vi "Update En Face Array.vi"(7 "State":T1, 8 "Error In":errorcluster, 9 "A-Scans Per B-Scan":u32, 10 "Number Of BScans":u32, 11 "Slice":sgl[](array[numeric])) -> (0 "Error Out":errorcluster, 2 "B-Scan Index":i32, 3 "Array out":sgl[][](array[numeric]))   [LabVIEW 2015, in "Intensity Processing.lvclass"]
uses:
  Intensity/Intensity Processing.lvclass
  En Face States.ctl
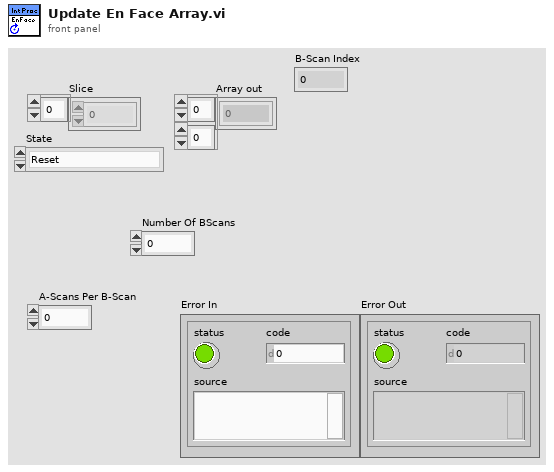
[diagram p1: front panel]
types:
  T1 = typedef "En Face States.ctl" = enum16{"Reset", "Update", "Get EnFace"}
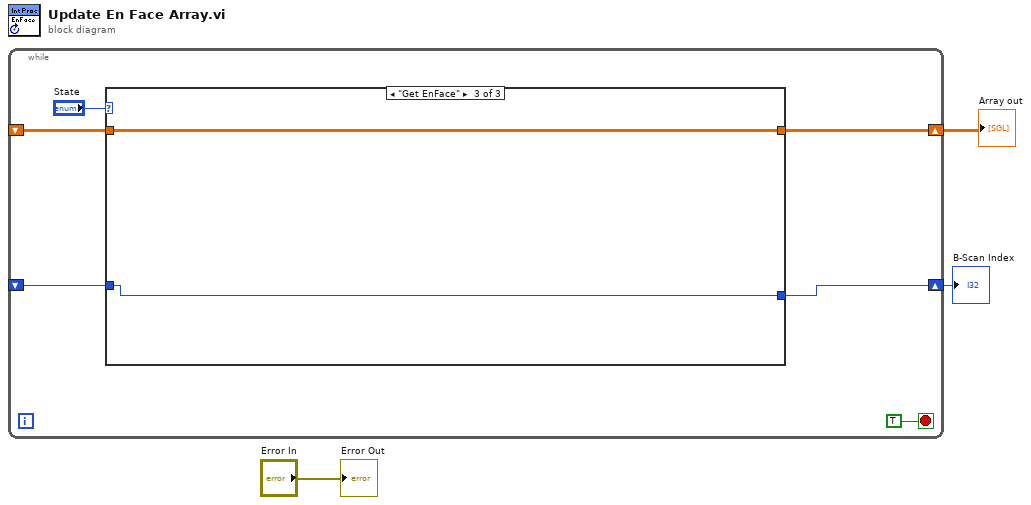
[diagram p0: block diagram]
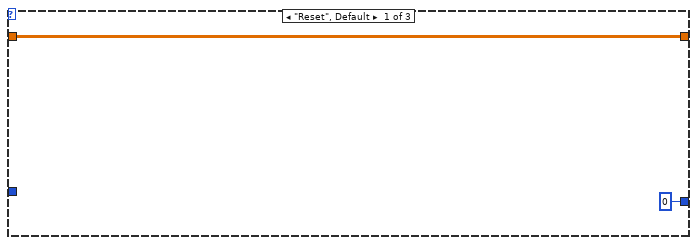
[diagram p2: hidden frame]
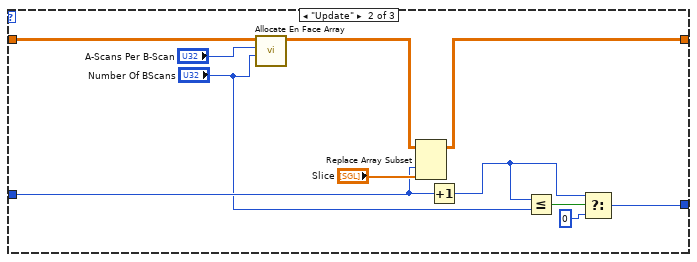
[diagram p3: hidden frame]
diagram:
  n1 = while {
    shift-right: [w8] -> w3
    shift-left: _ -> [w9]
    shift-right: [w6] -> w1
    shift-left: _ -> [w7]
    stop <- TRUE stop-if-true
    n2 = case shown="\"Get EnFace\"" "State" {
      tunnel: w9 -> [w10 w18 w24]
      tunnel: [w10 w17 w24] -> w8
      tunnel: w7 -> [_ w15 w23]
      tunnel: [0 ("f") w13 w23] -> w6
      frame "Reset", Default {
      }
      frame "Update" {
        n3 = call "Allocate En Face Array.vi"("Number of B-Scans"="Number Of BScans", "A-Scans Per B-Scan"="A-Scans Per B-Scan", ">> En Face Array >>"=w18) -> ("Array"=w19:sgl[][])  [unwired: 8 in]
        n4 = Replace Array Subset(array=w19, new element="Slice", index (col)=w15) -> (w17:sgl[][])  [unwired: 1 in]
        n5 = Increment(x=w15) -> (x+1=w14:i32)
        n6 = Less Or Equal?(x=w14, y="Number Of BScans") -> (x <= y?=w21:bool)
        n7 = Select(t=w14, s=w21, f=0) -> (s? t:f=w13:i32)
      }
      frame "Get EnFace" {
      }
    }
  }
  "Array out" <- w3
  "B-Scan Index" <- w1
  "Error Out" <- "Error In"
